vi "GetDatagroupName.vi"(8 "error in (no error)":errorcluster, 9 "Channels":T2[](array[typedef]), 10 "Properties":T1[](array[typedef])) -> (0 "error out":errorcluster, 3 "Data Group Name":string)   [LabVIEW 2017, in "McsaVirtualChannel.lvlib"]
uses:
  <vilib>/addons/InsightCM/Devices/Shared/Mcsa/McsaVirtualChannel/McsaVirtualChannel.lvlib
  <vilib>/addons/InsightCM/MessageBus/Base/controls/R2_Channel.ctl
  <vilib>/addons/InsightCM/MessageBus/Base/controls/KeyValuePair.ctl
  <vilib>/addons/InsightCM/MessageBus/Base/controls/Metric.ctl
  <vilib>/addons/InsightCM/Utilities/MCSA/McsaUtilities.lvlib
  <vilib>/addons/InsightCM/Utilities/PropertyHelpers/PropertyHelpers.lvlib
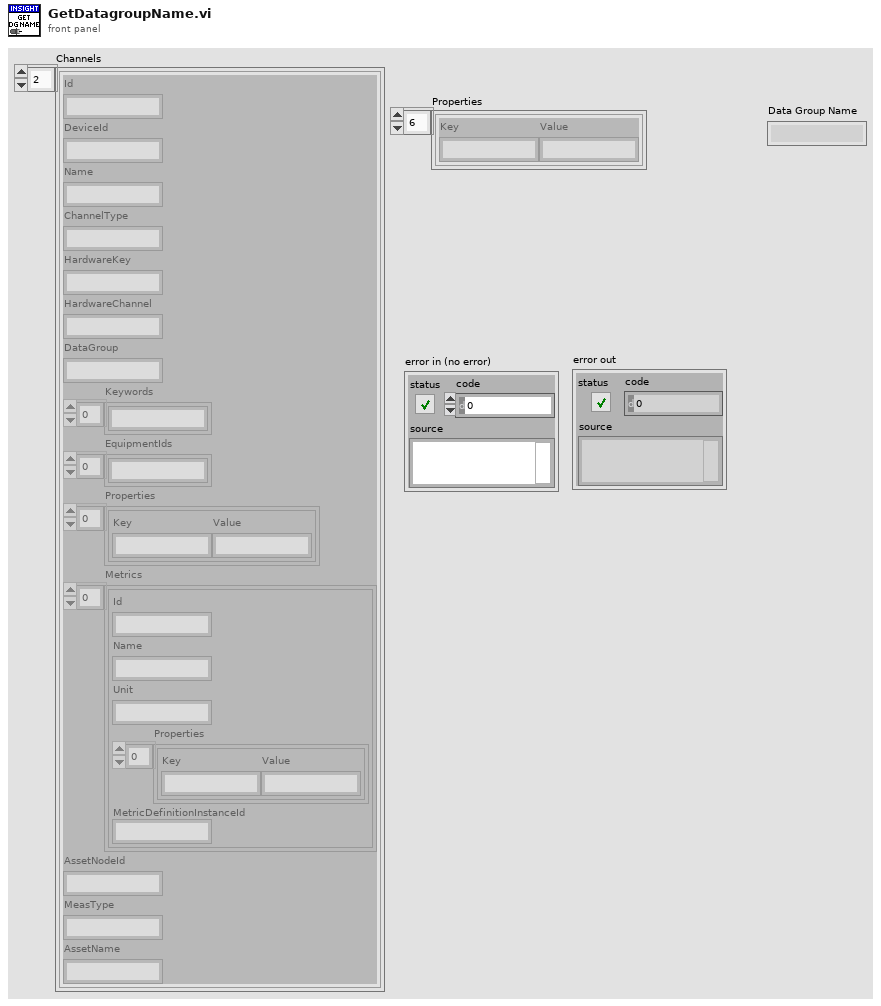
[diagram p1: front panel]
types:
  T1 = typedef "KeyValuePair.ctl" = cluster{"Key":string, "Value":string}
  T2 = typedef "R2_Channel.ctl" = cluster{"Id":string, "DeviceId":string, "Name":string, "ChannelType":string, "HardwareKey":string, "HardwareChannel":string, "DataGroup":string, "Keywords":string[], "EquipmentIds":string[], "Properties":T1[], "Metrics":T3[], "AssetNodeId":string, "MeasType":string, "AssetName":string}
  T3 = typedef "Metric.ctl" = cluster{"Id":string, "Name":string, "Unit":string, "Properties":T1[], "MetricDefinitionInstanceId":string}
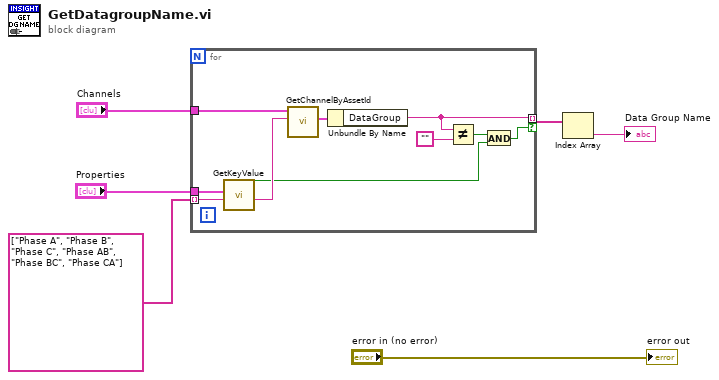
[diagram p0: block diagram]
diagram:
  n1 = for {
    tunnel: "Properties" -> [w16]
    tunnel: "Channels" -> [w15]
    tunnel: string[] ["Phase A", "Phase B", "Phase C", "Phase AB", "Phase BC", "Phase CA"] -> [w13] mode=indexing
    tunnel: [w11] -> w1 mode=indexing if=w7
    n2 = call <vilib>:"GetKeyValue.vi"("key"=w13, "key value pairs"=w16) -> ("value"=w14:string, "found"=w8:bool)  [unwired: 7 in, 1 out]
    n3 = call <vilib>:"GetChannelByAssetId.vi"("node id"=w14, "channels in"=w15) -> ("channel"=w12:T2)  [unwired: 7 in, 2 out]
    n4 = Unbundle By Name(w12) -> ("DataGroup"=w11:string)
    n5 = Not Equal?(x=w11, y="") -> (x != y?=w9:bool)
    n6 = And(x=w9, y=w8) -> (x .and. y?=w7:bool)
  }
  n7 = Index Array(array=w1) -> (element=→"Data Group Name":string)  [unwired: 1 in]
  "error out" <- "error in (no error)"
